vi "Periodic Tasks.vi"(8 "error in":errorcluster) -> ()   [LabVIEW 2017]
doc: "This VI runs in parallel to other tasks. It can contain as many user-defined periodic loops as you need. These can carry out PID or other sorts of timed response."
uses:
  <vilib>/Rock Robotics/WPI/Solenoid/WPI_SolenoidValue.ctl
  <vilib>/Rock Robotics/WPI/Relay/WPI_RelayValue.ctl
  <vilib>/Rock Robotics/WPI/Utilities/WPI_GetSetVariantRefNum.vi
  <vilib>/Rock Robotics/Network Tables/NT Write Boolean.vi
  Robot Global Data.vi
  <vilib>/Rock Robotics/WPI/ThirdParty/Phoenix-LabVIEW/Pigeon IMU/CTRE_PigeonIMU_GetRawGyro.vi
  <vilib>/Rock Robotics/Network Tables/NT Write Number.vi
  <vilib>/Rock Robotics/WPI/ThirdParty/Phoenix-LabVIEW/Pigeon IMU/CTRE_PigeonIMU_GetFusedHeading.vi
  <vilib>/Rock Robotics/WPI/ThirdParty/Phoenix-LabVIEW/Pigeon IMU/CTRE_PigeonIMU_GetYPR.vi
  <vilib>/Rock Robotics/WPI/ThirdParty/Phoenix-LabVIEW/Motor Controller/Get/CTRE_Phoenix_MotorController_GetLimitSwitchStates.vi
  <vilib>/Rock Robotics/WPI/ThirdParty/Phoenix-LabVIEW/Motor Controller/Get/CTRE_Phoenix_MotorController_GetSelectedSensorData.vi
  <vilib>/Rock Robotics/WPI/Solenoid/WPI_SolenoidSetEnum.vi
  <vilib>/Rock Robotics/Network Tables/NT Write Numeric Array.vi
  <vilib>/Rock Robotics/Network Tables/NT Write Boolean Array.vi
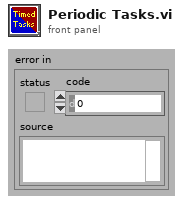
[diagram p1: front panel]
types:
  T1 = typedef "WPI_MotorControlDeviceRef.ctl" = cluster{"DeviceStatus":errorcluster, "Type":T2, "PWM":cluster{"PWM Channel":T3, "DeadBand":T4}, "CAN":cluster{"Device Number":u8, "SetOutput VI Ref":variant, "GetOutput VI Ref":variant, "Enable VI Ref":variant, "Disable VI Ref":variant, "Data":variant}, "Invert":bool, "DIO PWM":cluster{"PWM \"Enable\" Channel":T3, "DIOChannel":T5, "PWM Rate":dbl}}
  T2 = typedef "WPI_MotorControlType.ctl" = enum16{"PWM", "CAN", "DIO PWM"}
  T3 = typedef "FPGA_DIOPWMChannel.ctl" = enum8{"PWM 0", "PWM 1", "PWM 2", "PWM 3", "PWM 4", "PWM 5", "PWM 6", "PWM 7", "PWM 8", "PWM 9", "PWM MXP 0", "PWM MXP 1", "PWM MXP 2", "PWM MXP 3", "PWM MXP 4", "PWM MXP 5", "PWM MXP 6", "PWM MXP 7", "PWM MXP 8", "PWM MXP 9", "Invalid"}
  T4 = typedef "WPI_PWMDeadband.ctl" = cluster{"Name":string, "maxPositivePwm":i32, "minPositivePwm":i32, "centerPwm":i32, "maxNegativePwm":i32, "minNegativePwm":i32, "angularRange":u16}
  T5 = typedef "FPGA_DIOChannel.ctl" = enum8{"DIO 0", "DIO 1", "DIO 2", "DIO 3", "DIO 4", "DIO 5", "DIO 6", "DIO 7", "DIO 8", "DIO 9", "DIO MXP 0", "DIO MXP 1", "DIO MXP 2", "DIO MXP 3", "DIO MXP 4", "DIO MXP 5", "DIO MXP 6", "DIO MXP 7", "DIO MXP 8", "DIO MXP 9", "DIO MXP 10", "DIO MXP 11", "DIO MXP 12", "DIO MXP 13", "DIO MXP 14", "DIO MXP 15", "SPI Port CS1", "SPI Port CS2", "SPI Port CS3", "SPI Port MISO", "SPI Port MOSI", "Invalid"}
  T6 = typedef "WPI_AnalogChannelDevRef.ctl" = cluster{"DevStatus":errorcluster, "Analog Channel":T7}
  T7 = typedef "FPGA_AIChannel.ctl" = enum8{"AI 0", "AI 1", "AI 2", "AI 3", "AI MXP 0", "AI MXP 1", "AI MXP 2", "AI MXP 3", "Invalid"}
  T8 = typedef "WPI_RelayValue.ctl" = enum16{"Off", "On", "Forward", "Reverse"}
  T9 = typedef "CTRE_PigeonIMU_DeviceRef.ctl" = cluster{"DeviceStatus":errorcluster, "Device Number":u8, "Type":T10, "Device ID":u32, "Handle":u64, "UsageFrame":u32, "Library Path":path}
  T10 = typedef "CTRE_PigeonIMU_ConnectionType.ctl" = u32
  T11 = typedef "WPI_CompressorDevRef.ctl" = cluster{"DevStatus":errorcluster, "Pneumatics Control Module":u8}
  T12 = typedef "WPI_RelayDevRef.ctl" = cluster{"DevStatus":errorcluster, "Relay Channel":T13, "Relay Direction":T14}
  T13 = typedef "FPGA_DIORelayChannel.ctl" = enum8{"Relay 0", "Relay 1", "Relay 2", "Relay 3", "Invalid"}
  T14 = typedef "WPI_RelayDirection.ctl" = enum16{"Both directions", "Forward only", "Reverse only"}
  T15 = cluster{"Heading":dbl, "Valid?":bool, "Fusing?":bool}
  T16 = cluster{"X":dbl, "Y":dbl, "Z":dbl, "Magnitude":dbl}
  T17 = typedef "WPI_DriverStationRobotMode2.ctl" = enum16{"Autonomous Disabled", "Autonomous Enabled", "Teleop Disabled", "Teleop Enabled", "Disconnected", "Finish", "Test Disabled", "Test Enabled", "Emergency Stopped"}
  T18 = typedef "WPI_SolenoidValue.ctl" = enum16{"Off", "On", "Forward", "Reverse"}
  T19 = typedef "WPI_SolenoidDevRef.ctl" = cluster{"DevStatus":errorcluster, "Pneumatics Control Module":u8, "Forward Solenoid Channel":T20, "Reverse Solenoid Channel":T20}
  T20 = typedef "WPI_SolenoidChannel.ctl" = enum8{"Solenoid 0", "Solenoid 1", "Solenoid 2", "Solenoid 3", "Solenoid 4", "Solenoid 5", "Solenoid 6", "Solenoid 7", "Invalid"}
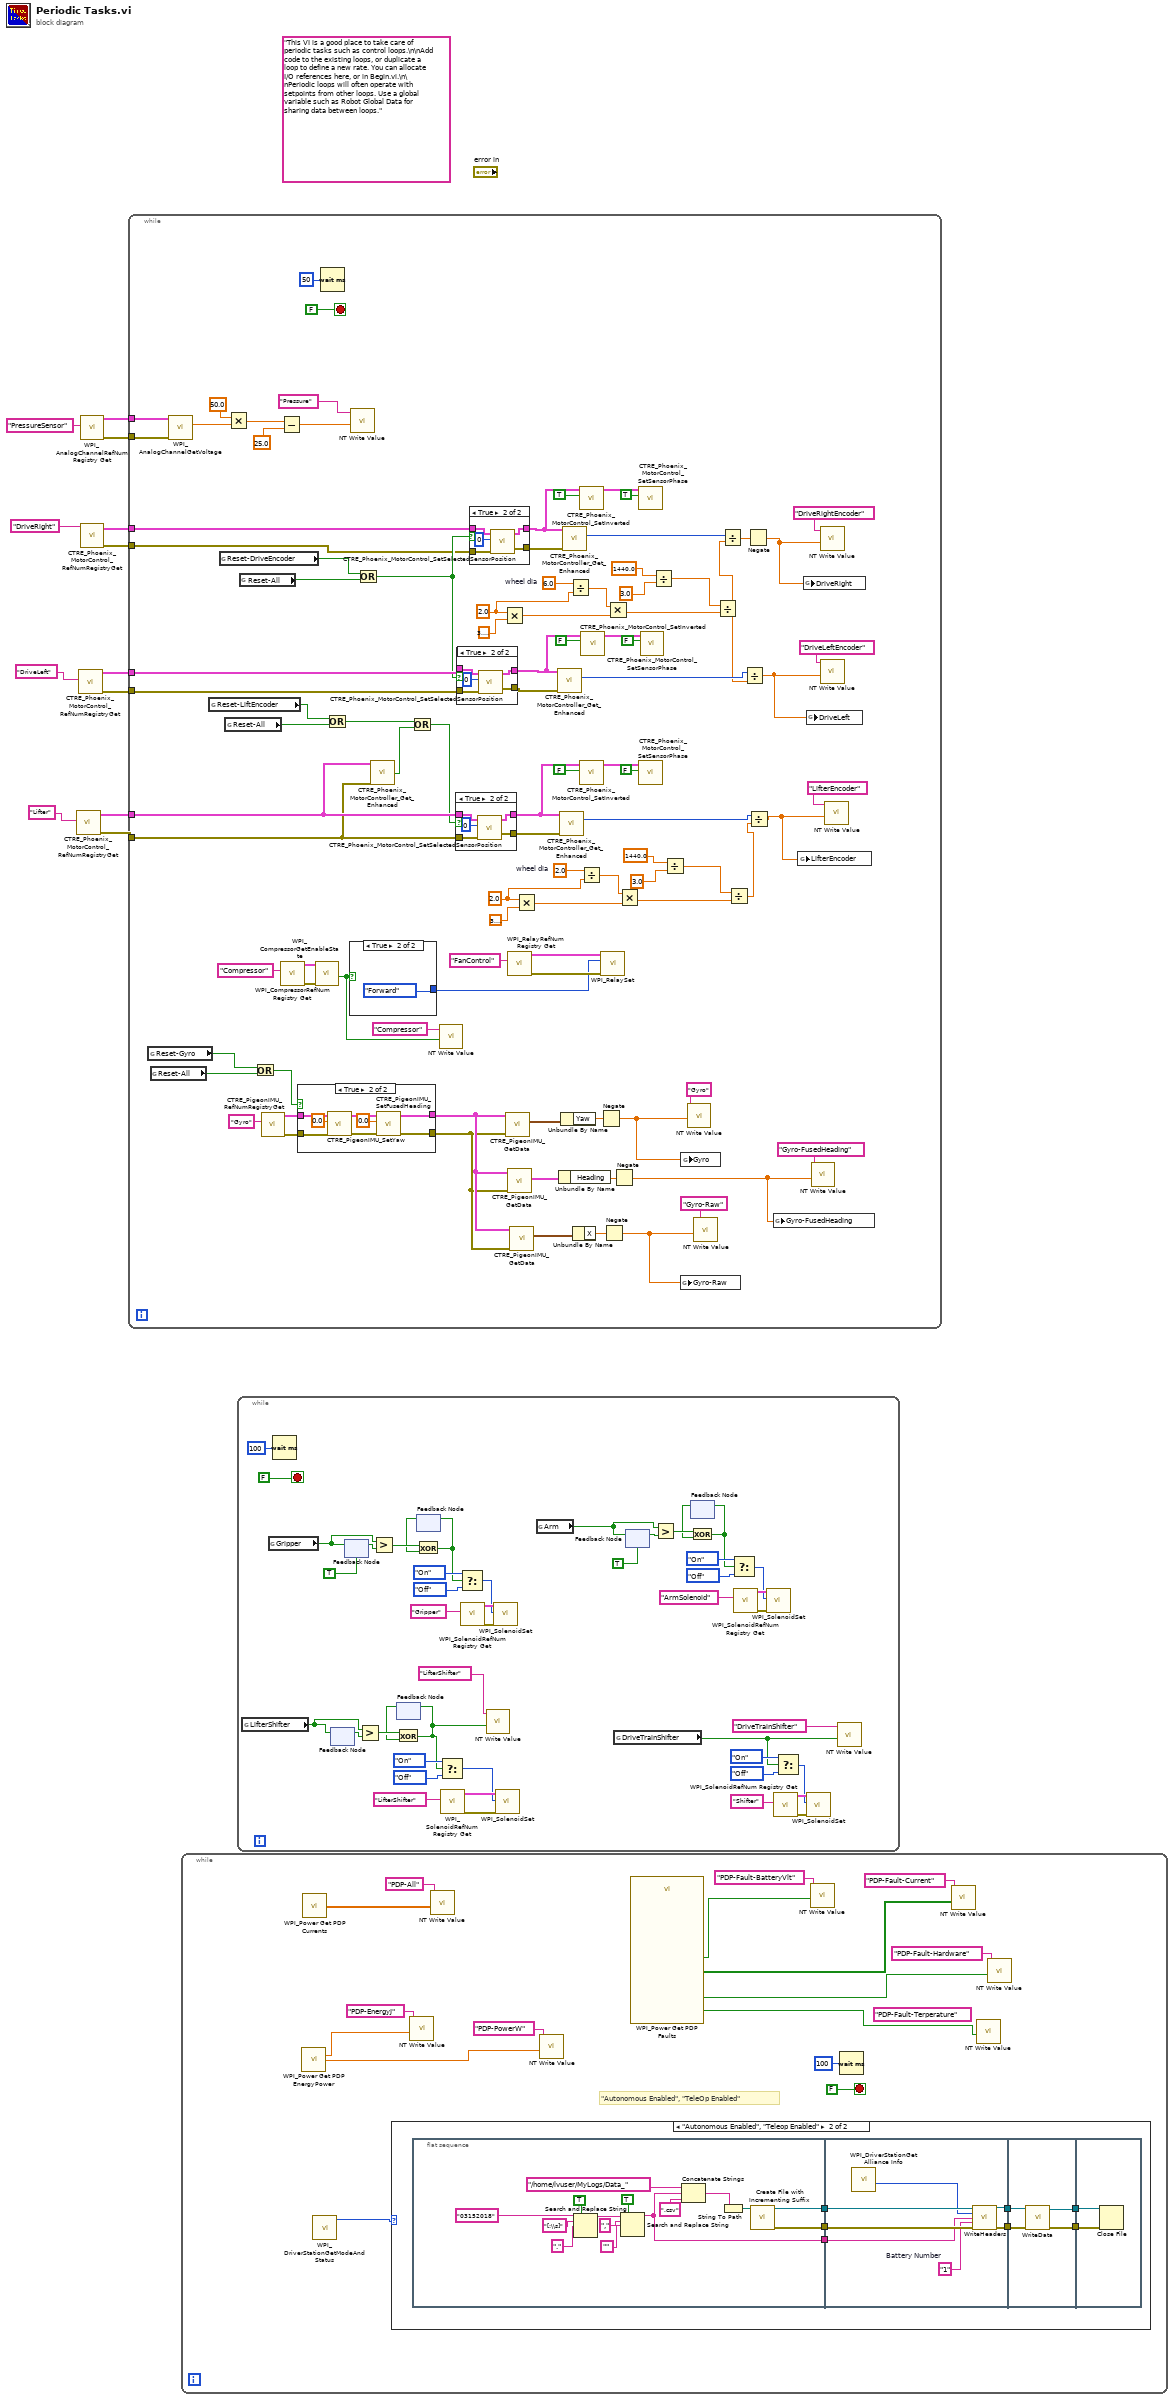
[diagram p0: block diagram]
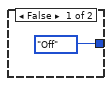
[diagram p3: hidden frame]
diagram:
  (unwired) "This VI is a good place to take care of periodic tasks such as control loops.\n\nAdd code to the existing loops, or duplicate a loop to define a new rate. You can allocate I/O references here, or in Begin.vi.\n\nPeriodic loops will often operate with setpoints from other loops. Use a global variable such as Robot Global Data for sharing data between loops."
  n1 = call <vilib>:"CTRE_Phoenix_MotorControl_RefNumRegistryGet.vi"("refnum name"="Lifter") -> ("error out"=w6:errorcluster, "PhoenixMotorControlDevRef"=w7:T1)  [unwired: 9 in]
  n2 = call <vilib>:"CTRE_Phoenix_MotorControl_RefNumRegistryGet.vi"("refnum name"="DriveLeft") -> ("error out"=w5:errorcluster, "PhoenixMotorControlDevRef"=w9:T1)  [unwired: 9 in]
  n3 = call <vilib>:"WPI_AnalogChannelRefNum Registry Get.vi"("refnum name"="PressureSensor") -> ("error out"=w1:errorcluster, "AIDeviceRef"=w2:T6)  [unwired: 9 in]
  n4 = call <vilib>:"CTRE_Phoenix_MotorControl_RefNumRegistryGet.vi"("refnum name"="DriveRight") -> ("error out"=w4:errorcluster, "PhoenixMotorControlDevRef"=w11:T1)  [unwired: 9 in]
  n5 = while {
    tunnel: w11 -> [w83]
    tunnel: w9 -> [w84]
    tunnel: w7 -> [w26]
    tunnel: w6 -> [w25]
    tunnel: w5 -> [w81]
    tunnel: w4 -> [w80]
    tunnel: w2 -> [w22]
    tunnel: w1 -> [w21]
    stop <- FALSE stop-if-true
    w63 = 2.0
    w64 = 2.0  # wheel dia
    w77 = 2.0
    w78 = 6.0  # wheel dia
    n6 = global read "Robot Global Data.vi" "Reset-Gyro"() -> (w88:bool)
    n7 = global read "Robot Global Data.vi" "Reset-All"() -> (w89:bool)
    n8 = call <vilib>:"WPI_AnalogChannelGetVoltage.vi"("error in (no error)"=w21, "AIDeviceRef"=w22) -> ("Voltage"=w15:dbl)  [unwired: 7 in, 2 out]
    n9 = global read "Robot Global Data.vi" "Reset-LiftEncoder"() -> (w86:bool)
    n10 = global read "Robot Global Data.vi" "Reset-DriveEncoder"() -> (w90:bool)
    n11 = global read "Robot Global Data.vi" "Reset-All"() -> (w87:bool)
    n12 = Multiply(x=50.0, y=w15) -> (x*y=w19:dbl)
    n13 = global read "Robot Global Data.vi" "Reset-All"() -> (w99:bool)
    n14 = Or(x=w88, y=w89) -> (x .or. y?=w52:bool)
    n15 = call <vilib>:"CTRE_PigeonIMU_RefNumRegistryGet.vi"("refnum name"="Gyro") -> ("error out"=w97:errorcluster, "PigeonIMUDevRef"=w98:T9)  [unwired: 9 in]
    n16 = Subtract(x=w19, y=25.0) -> (x-y=w17:dbl)
    n17 = call <vilib>:"WPI_CompressorRefNum Registry Get.vi"("refnum name"="Compressor") -> ("error out"=w93:errorcluster, "CompressorDevRef"=w92:T11)  [unwired: 9 in]
    n18 = case shown="True" w52 {
      tunnel: w98 -> [w114 w121]
      tunnel: [w114 w116] -> w33
      tunnel: w97 -> [w113 w119]
      tunnel: [w113 w118] -> w32
      frame False {
      }
      frame True {
        n19 = call <vilib>:"CTRE_PigeonIMU_SetYaw.vi"("error in (no error)"=w119, "Value"=0.0, "PigeonIMUDevRef"=w121) -> ("error out"=w118:errorcluster, "PigeonIMUDevRef"=w120:T9)  [unwired: 7 in]
        n20 = call <vilib>:"CTRE_PigeonIMU_SetFusedHeading.vi"("Value"=0.0, "PigeonIMUDevRef 2"=w120) -> ("PigeonIMUDevRef"=w116:T9)  [unwired: 8 in, 1 out]
      }
    }
    n21 = call <vilib>:"WPI_CompressorGetEnableState.vi"("error in (no error)"=w93, "CompressorDevRef"=w92) -> ("Compressor Running"=w14:bool)  [unwired: 6 in, 3 out]
    n22 = Wait (ms)(milliseconds to wait=u32 50) -> ()  [unwired: 1 out]
    n23 = Or(x=w86, y=w87) -> (x .or. y?=w85:bool)
    n24 = case shown="True" w14 {
      tunnel: [WPI_RelayValue."Off" ("RelayValue") WPI_RelayValue."Forward" ("RelayValue")] -> w94
      frame False {
      }
      frame True {
      }
    }
    n25 = call-poly <vilib>:"NT Write Value.vi"("Numeric"=w17, "Name"="Pressure") -> ()  [unwired: 9 in, 1 out]
    n26 = Or(x=w90, y=w99) -> (x .or. y?=w82:bool)
    n27 = call-poly <vilib>:"CTRE_Phoenix_MotorController_Get_Enhanced.vi"("PhoenixMotorControlDevRef"=w26, "error in"=w25) -> ("Reverse Limit Closed?"=w23:bool)  [unwired: 10 in, 3 out]
    n28 = Or(x=w85, y=w23) -> (x .or. y?=w24:bool)
    n29 = call-poly <vilib>:"NT Write Value.vi"("Boolean"=w14, "Name"="Compressor") -> ()  [unwired: 9 in, 1 out]
    n30 = case shown="True" w24 {
      tunnel: w26 -> [w137 w142]
      tunnel: [w137 w141] -> w38
      tunnel: [w136 w140] -> w102
      tunnel: w25 -> [w136 w138]
      frame False {
      }
      frame True {
        n31 = call <vilib>:"CTRE_Phoenix_MotorControl_SetSelectedSensorPosition.vi"("error in (no error)"=w138, "New Sensor Position"=0, "PhoenixMotorControlDevRef"=w142) -> ("error out"=w140:errorcluster, "PhoenixMotorControlDevRef"=w141:T1)  [unwired: 7 in]
      }
    }
    n32 = case shown="True" w82 {
      tunnel: w84 -> [w130 w135]
      tunnel: [w129 w134] -> w101
      tunnel: [w130 w132] -> w42
      tunnel: w81 -> [w129 w131]
      frame False {
      }
      frame True {
        n33 = call <vilib>:"CTRE_Phoenix_MotorControl_SetSelectedSensorPosition.vi"("error in (no error)"=w131, "New Sensor Position"=0, "PhoenixMotorControlDevRef"=w135) -> ("error out"=w134:errorcluster, "PhoenixMotorControlDevRef"=w132:T1)  [unwired: 7 in]
      }
    }
    n34 = case shown="True" w82 {
      tunnel: w83 -> [w123 w128]
      tunnel: [w123 w127] -> w48
      tunnel: [w122 w126] -> w100
      tunnel: w80 -> [w122 w124]
      frame False {
      }
      frame True {
        n35 = call <vilib>:"CTRE_Phoenix_MotorControl_SetSelectedSensorPosition.vi"("error in (no error)"=w124, "New Sensor Position"=0, "PhoenixMotorControlDevRef"=w128) -> ("error out"=w126:errorcluster, "PhoenixMotorControlDevRef"=w127:T1)  [unwired: 7 in]
      }
    }
    n36 = Multiply(x=w77, y=3.141592653589793) -> (x*y=w75:dbl)
    n37 = call-poly <vilib>:"CTRE_PigeonIMU_GetData.vi"("error in (no error)"=w32, "PigeonIMUDevRef"=w33) -> ("Yaw Pitch Roll"=w108:cluster{"Yaw":dbl, "Pitch":dbl, "Roll":dbl})  [unwired: 7 in, 2 out]
    n38 = call <vilib>:"WPI_RelayRefNum Registry Get.vi"("refnum name"="FanControl") -> ("error out"=w95:errorcluster, "RelayDevRef"=w27:T12)  [unwired: 9 in]
    n39 = call-poly <vilib>:"CTRE_PigeonIMU_GetData.vi"("error in (no error)"=w32, "PigeonIMUDevRef"=w33) -> ("Fused Heading"=w36:T15)  [unwired: 7 in, 2 out]
    n40 = call-poly <vilib>:"CTRE_PigeonIMU_GetData.vi"("error in (no error)"=w32, "PigeonIMUDevRef"=w33) -> ("Gyro DPS"=w31:T16)  [unwired: 7 in, 2 out]
    n41 = Multiply(x=w63, y=3.141592653589793) -> (x*y=w61:dbl)
    n42 = call-poly <vilib>:"CTRE_Phoenix_MotorController_Get_Enhanced.vi"("PhoenixMotorControlDevRef"=w42, "error in"=w101) -> ("Position (Raw Sensor Units)"=w67:i32)  [unwired: 10 in, 3 out]
    n43 = Unbundle By Name(w36) -> ("Heading"=w35:dbl)
    n44 = call-poly <vilib>:"CTRE_Phoenix_MotorController_Get_Enhanced.vi"("PhoenixMotorControlDevRef"=w38, "error in"=w102) -> ("Position (Raw Sensor Units)"=w56:i32)  [unwired: 10 in, 3 out]
    n45 = Unbundle By Name(w108) -> ("Yaw"=w51:dbl)
    n46 = call-poly <vilib>:"CTRE_Phoenix_MotorController_Get_Enhanced.vi"("PhoenixMotorControlDevRef"=w48, "error in"=w100) -> ("Position (Raw Sensor Units)"=w70:i32)  [unwired: 10 in, 3 out]
    n47 = Divide(x=w78, y=w77) -> (x/y=w76:dbl)
    n48 = Unbundle By Name(w31) -> ("X"=w29:dbl)
    n49 = call <vilib>:"CTRE_Phoenix_MotorControl_SetInverted.vi"("Invert?"=TRUE, "PhoenixMotorControlDevRef"=w48) -> ("PhoenixMotorControlDevRef"=w49:T1)  [unwired: 8 in, 1 out]
    n50 = call <vilib>:"CTRE_Phoenix_MotorControl_SetInverted.vi"("Invert?"=FALSE, "PhoenixMotorControlDevRef"=w38) -> ("PhoenixMotorControlDevRef"=w41:T1)  [unwired: 8 in, 1 out]
    n51 = Divide(x=w64, y=w63) -> (x/y=w62:dbl)
    n52 = call <vilib>:"CTRE_Phoenix_MotorControl_SetInverted.vi"("Invert?"=FALSE, "PhoenixMotorControlDevRef"=w42) -> ("PhoenixMotorControlDevRef"=w45:T1)  [unwired: 8 in, 1 out]
    n53 = Negate(x=w51) -> (-x=w50:dbl)
    n54 = call <vilib>:"WPI_RelaySet.vi"("error in (no error)"=w95, "RelayValue"=w94, "RelayDevRef"=w27) -> ()  [unwired: 7 in, 2 out]
    n55 = Negate(x=w29) -> (-x=w28:dbl)
    n56 = Multiply(x=w76, y=w75) -> (x*y=w74:dbl)
    n57 = Negate(x=w35) -> (-x=w34:dbl)
    n58 = Multiply(x=w62, y=w61) -> (x*y=w60:dbl)
    n59 = call <vilib>:"CTRE_Phoenix_MotorControl_SetSensorPhase.vi"("PhaseSensor"=TRUE, "PhoenixMotorControlDevRef"=w49) -> ()  [unwired: 8 in, 2 out]
    n60 = call <vilib>:"CTRE_Phoenix_MotorControl_SetSensorPhase.vi"("PhaseSensor"=FALSE, "PhoenixMotorControlDevRef"=w41) -> ()  [unwired: 8 in, 2 out]
    n61 = call <vilib>:"CTRE_Phoenix_MotorControl_SetSensorPhase.vi"("PhaseSensor"=FALSE, "PhoenixMotorControlDevRef"=w45) -> ()  [unwired: 8 in, 2 out]
    n62 = Divide(x=1440.0, y=3.0) -> (x/y=w71:dbl)
    n63 = Divide(x=1440.0, y=3.0) -> (x/y=w58:dbl)
    n64 = global write "Robot Global Data.vi" "Gyro-Raw"(w28) -> ()
    n65 = global write "Robot Global Data.vi" "Gyro"(w50) -> ()
    n66 = call-poly <vilib>:"NT Write Value.vi"("Numeric"=w50, "Name"="Gyro") -> ()  [unwired: 9 in, 1 out]
    n67 = call-poly <vilib>:"NT Write Value.vi"("Numeric"=w28, "Name"="Gyro-Raw") -> ()  [unwired: 9 in, 1 out]
    n68 = Divide(x=w71, y=w74) -> (x/y=w66:dbl)
    n69 = Divide(x=w70, y=w66) -> (x/y=w69:dbl)
    n70 = Divide(x=w58, y=w60) -> (x/y=w54:dbl)
    n71 = Divide(x=w67, y=w66) -> (x/y=w68:dbl)
    n72 = Negate(x=w69) -> (-x=w53:dbl)
    n73 = Divide(x=w56, y=w54) -> (x/y=w55:dbl)
    n74 = global write "Robot Global Data.vi" "Gyro-FusedHeading"(w34) -> ()
    n75 = global write "Robot Global Data.vi" "LifterEncoder"(w55) -> ()
    n76 = global write "Robot Global Data.vi" "DriveRight"(w53) -> ()
    n77 = global write "Robot Global Data.vi" "DriveLeft"(w68) -> ()
    n78 = call-poly <vilib>:"NT Write Value.vi"("Numeric"=w34, "Name"="Gyro-FusedHeading") -> ()  [unwired: 9 in, 1 out]
    n79 = call-poly <vilib>:"NT Write Value.vi"("Numeric"=w53, "Name"="DriveRightEncoder") -> ()  [unwired: 9 in, 1 out]
    n80 = call-poly <vilib>:"NT Write Value.vi"("Numeric"=w68, "Name"="DriveLeftEncoder") -> ()  [unwired: 9 in, 1 out]
    n81 = call-poly <vilib>:"NT Write Value.vi"("Numeric"=w55, "Name"="LifterEncoder") -> ()  [unwired: 9 in, 1 out]
  }
  n82 = while {
    stop <- FALSE stop-if-true
    (unwired) "PDP-Fault-Terperature" ("Name")
    # "\"Autonomous Enabled\", \"TeleOp Enabled\""
    n83 = call <vilib>:"WPI_Power Get PDP EnergyPower.vi"() -> ("Energy (J)"=w153:dbl, "Power (W)"=w151:dbl)  [unwired: 13 in, 1 out]
    n84 = call <vilib>:"WPI_Power Get PDP Currents.vi"() -> ("all currents (A)"=w155:dbl[])  [unwired: 13 in, 2 out]
    n85 = call <vilib>:"WPI_DriverStationGetModeAndStatus.vi"() -> ("Robot Mode"=w150:T17)  [unwired: 10 in, 1 out]
    n86 = case shown="\"Autonomous Enabled\", \"Teleop Enabled\"" w150 {
      frame Default {
        # "Logging turned off\nRobot is not enabled"
      }
      frame "Autonomous Enabled", "Teleop Enabled" {
        n87 = flat-sequence {
          tunnel: [w167] -> w165
          tunnel: [w168] -> w164
          tunnel: [w176] -> w163
          tunnel: w165 -> [w184]
          tunnel: w164 -> [w183]
          tunnel: w163 -> [w185]
          tunnel: [w187] -> w162
          tunnel: [w186] -> w161
          tunnel: w162 -> [w191]
          tunnel: [w188] -> w160
          tunnel: [w189] -> w159
          tunnel: w161 -> [w190]
          tunnel: w160 -> [w193]
          tunnel: w159 -> [w192]
          frame #0 {
            n88 = Search and Replace String(replace all?=TRUE ("replace all? (F)"), input string="03152018", search string="[:\\s]", replace string="." ("replace string (\"\")")) -> (result string=w172:string)  [unwired: 4 in, 3 out]
            n89 = Search and Replace String(replace all?=TRUE ("replace all? (F)"), input string=w172, search string=",", replace string="") -> (result string=w168:string)  [unwired: 4 in, 3 out]
            n90 = Concatenate Strings("/home/lvuser/MyLogs/Data_" ("string"), w168, ".csv" ("string")) -> (w178:string)
            n91 = String To Path(string=w178) -> (path=w177:path)
            n92 = call <vilib>:"Create File with Incrementing Suffix.vi"("file path"=w177) -> ("error out"=w176:errorcluster, "refnum out"=w167:refnum<file>)  [unwired: 8 in, 1 out]
          }
          frame #1 {
            w182 = "1"  # Battery Number
            n93 = call <vilib>:"WPI_DriverStationGet Alliance Info.vi"() -> ("Match Number"=w181:u16)  [unwired: 6 in, 5 out]
            n94 = call "WriteHeaders.vi"("refnum in"=w184, "Match Number"=w181, "Date and Time"=w183, "Battery Number"=w182, "error in"=w185) -> ("refnum out"=w187:refnum<file>, "error out"=w186:errorcluster)  [unwired: 9 in]
          }
          frame #2 {
            n95 = call "WriteData.vi"("error in"=w190, "refnum in"=w191) -> ("error out"=w189:errorcluster, "refnum out"=w188:refnum<file>)  [unwired: 8 in]
          }
          frame #3 {
            n96 = Close File(refnum=w193, error in=w192) -> ()  [unwired: 2 out]
          }
        }
      }
    }
    n97 = call-poly <vilib>:"NT Write Value.vi"("Numeric"=w153, "Name"="PDP-EnergyJ") -> ()  [unwired: 9 in, 1 out]
    n98 = call-poly <vilib>:"NT Write Value.vi"("Numeric Array"=w155, "Name"="PDP-All") -> ()  [unwired: 9 in, 1 out]
    n99 = call-poly <vilib>:"NT Write Value.vi"("Numeric"=w151, "Name"="PDP-PowerW") -> ()  [unwired: 9 in, 1 out]
    n100 = call <vilib>:"WPI_Power Get PDP Faults.vi"() -> ("Current Faults"=w146:bool[], "Battery Voltage Fault"=w148:bool, "Temperature Fault"=w143:bool, "Hardware Fault"=w144:bool)  [unwired: 11 in, 1 out]
    n101 = call-poly <vilib>:"NT Write Value.vi"("Boolean"=w148, "Name"="PDP-Fault-BatteryVlt") -> ()  [unwired: 9 in, 1 out]
    n102 = Wait (ms)(milliseconds to wait=u32 100) -> ()  [unwired: 1 out]
    n103 = call-poly <vilib>:"NT Write Value.vi"("Boolean Array"=w146, "Name"="PDP-Fault-Current") -> ()  [unwired: 9 in, 1 out]
    n104 = call-poly <vilib>:"NT Write Value.vi"("Boolean"=w143) -> ()  [unwired: 10 in, 1 out]
    n105 = call-poly <vilib>:"NT Write Value.vi"("Boolean"=w144, "Name"="PDP-Fault-Hardware") -> ()  [unwired: 9 in, 1 out]
  }
  n106 = while {
    stop <- FALSE stop-if-true
    n107 = global read "Robot Global Data.vi" "LifterShifter"() -> (w202:bool)
    n108 = global read "Robot Global Data.vi" "Gripper"() -> (w227:bool)
    n109 = Wait (ms)(milliseconds to wait=u32 100) -> ()  [unwired: 1 out]
    n110 = feedback #1() -> (w210:bool)  [unwired: 1 in]
    n111 = feedback-in #1(w202) -> ()
    n112 = feedback #2(TRUE ("Gripper")) -> (w234:bool)
    n113 = feedback-in #2(w227) -> ()
    n114 = Greater?(x=w202, y=w210) -> (0:w209:bool)
    n115 = Greater?(x=w227, y=w234) -> (0:w233:bool)
    n116 = feedback #3() -> (w208:bool)  [unwired: 1 in]
    n117 = Exclusive Or(1:w208, 2:w209) -> (0:w203:bool)
    n118 = feedback-in #3(w203) -> ()
    n119 = feedback #4() -> (w232:bool)  [unwired: 1 in]
    n120 = Exclusive Or(1:w232, 2:w233) -> (0:w229:bool)
    n121 = feedback-in #4(w229) -> ()
    n122 = Select(t=WPI_SolenoidValue."On" ("Value"), s=w203, f=WPI_SolenoidValue."Off" ("Value")) -> (s? t:f=w205:T18)
    n123 = call <vilib>:"WPI_SolenoidRefNum Registry Get.vi"("refnum name"="LifterShifter") -> ("error out"=w212:errorcluster, "SolenoidDevRef"=w211:T19)  [unwired: 9 in]
    n124 = Select(t=WPI_SolenoidValue."On" ("Value"), s=w229, f=WPI_SolenoidValue."Off" ("Value")) -> (s? t:f=w228:T18)
    n125 = call <vilib>:"WPI_SolenoidRefNum Registry Get.vi"("refnum name"="Gripper") -> ("error out"=w236:errorcluster, "SolenoidDevRef"=w235:T19)  [unwired: 9 in]
    n126 = call-poly <vilib>:"NT Write Value.vi"("Boolean"=w203, "Name"="LifterShifter") -> ()  [unwired: 9 in, 1 out]
    n127 = call-poly <vilib>:"WPI_SolenoidSet.vi"("error in (no error)"=w236, "Value"=w228, "SolenoidDevRef"=w235) -> ()  [unwired: 7 in, 2 out]
    n128 = call-poly <vilib>:"WPI_SolenoidSet.vi"("error in (no error)"=w212, "Value"=w205, "SolenoidDevRef"=w211) -> ()  [unwired: 7 in, 2 out]
    n129 = global read "Robot Global Data.vi" "Arm"() -> (w216:bool)
    n130 = global read "Robot Global Data.vi" "DriveTrainShifter"() -> (w194:bool)
    n131 = feedback #5(TRUE ("Arm")) -> (w217:bool)
    n132 = feedback-in #5(w216) -> ()
    n133 = Greater?(x=w216, y=w217) -> (0:w223:bool)
    n134 = feedback #6() -> (w222:bool)  [unwired: 1 in]
    n135 = Exclusive Or(1:w222, 2:w223) -> (0:w219:bool)
    n136 = feedback-in #6(w219) -> ()
    n137 = Select(t=WPI_SolenoidValue."On" ("Value"), s=w219, f=WPI_SolenoidValue."Off" ("Value")) -> (s? t:f=w218:T18)
    n138 = call <vilib>:"WPI_SolenoidRefNum Registry Get.vi"("refnum name"="ArmSolenoid") -> ("error out"=w225:errorcluster, "SolenoidDevRef"=w224:T19)  [unwired: 9 in]
    n139 = call-poly <vilib>:"WPI_SolenoidSet.vi"("error in (no error)"=w225, "Value"=w218, "SolenoidDevRef"=w224) -> ()  [unwired: 7 in, 2 out]
    n140 = call <vilib>:"WPI_SolenoidRefNum Registry Get.vi"("refnum name"="Shifter") -> ("error out"=w200:errorcluster, "SolenoidDevRef"=w199:T19)  [unwired: 9 in]
    n141 = Select(t=WPI_SolenoidValue."On" ("Value"), s=w194, f=WPI_SolenoidValue."Off" ("Value")) -> (s? t:f=w196:T18)
    n142 = call-poly <vilib>:"WPI_SolenoidSet.vi"("error in (no error)"=w200, "Value"=w196, "SolenoidDevRef"=w199) -> ()  [unwired: 7 in, 2 out]
    n143 = call-poly <vilib>:"NT Write Value.vi"("Boolean"=w194, "Name"="DriveTrainShifter") -> ()  [unwired: 9 in, 1 out]
  }
